vi "Handle Last Ack Core.vi"(4 "error in (no error)":errorcluster, 6 "Last Ack":refnum<class "Last Ack.lvclass">, 7 "System Actor in":refnum<class "System Actor.lvclass">) -> (0 "error out":errorcluster, 3 "System Actor out":refnum<class "System Actor.lvclass">)   [LabVIEW 2013, in "Robot Actors.lvlib" / "System Actor.lvlib" / "System Actor.lvclass"]
doc: "(<B>Filename</B>: Actor Framework.lvlib:Actor.lvclass:Handle Last Ack Core.vi)\n\nDefines how the caller actor responds to the Last Ack message from a nested actor. The Last Ack message is the final message a nested actor sends to its caller before it shuts down. The message contains information about the final state of the nested actor.\n\nBy default, this method does nothing except return any error the nested actor sent. A descendant class may override this method to define behavior."
uses:
  System Actor.lvclass
  <vilib>/ActorFramework/LastAck/Last Ack.lvclass
  <vilib>/ActorFramework/LastAck/Last Ack.lvclass/Last Ack.ctl
  State Actor/State Actor.lvclass
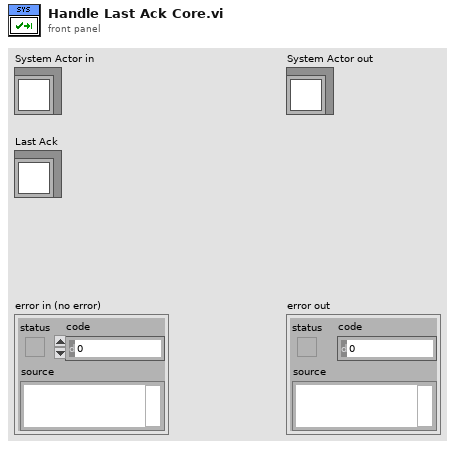
[diagram p1: front panel]
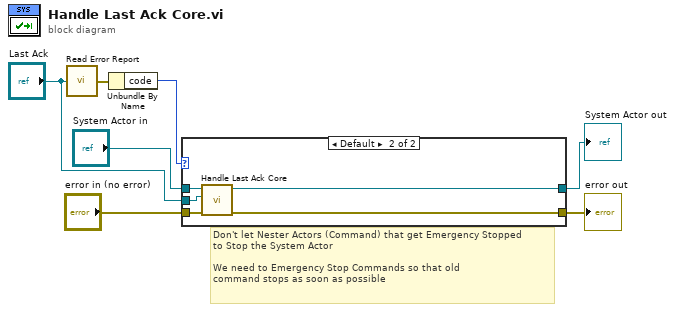
[diagram p0: block diagram]
diagram:
  # "Don't let Nester Actors (Command) that get Emergency Stopped\nto Stop the System Actor\n\nWe need to Emergency Stop Commands so that old\ncommand stops as soon as possible"
  n1 = call <vilib>:"Read Error Report.vi"("Last Ack"="Last Ack") -> ("error report"=w7:errorcluster)
  n2 = Unbundle By Name(w7) -> ("code"=w6:i32)
  n3 = case shown="Default" w6 {
    tunnel: "System Actor in" -> [w8 w14]
    tunnel: [w8 w13] -> w4
    tunnel: "error in (no error)" -> [w9 w12]
    tunnel: [w9 w11] -> w2
    tunnel: "Last Ack" -> [_ w10]
    frame 1608 {
      # "Don't Pass Up\nError on Emergency\nStop of Command"
    }
    frame Default {
      n4 = call-parent "Handle Last Ack Core.vi"("error in (no error)"=w12, "Last Ack"=w10, "Actor in"=w14) -> ("error out"=w11:errorcluster, "Actor out"=w13:refnum<class "System Actor.lvclass">)  [unwired: 3 in]
    }
  }
  "System Actor out" <- w4
  "error out" <- w2
